vi "02.Evd.2_Ask.2.vi"() -> ()   [LabVIEW 2025]
panel:
  in  "Initial temperature in °C":dbl
  out "Kelvin":dbl
  out "Celsius":dbl
  out "Fahrenheit":dbl
  out "Kelvin":dbl(slide) scale=0.0..500.0
  out "Celsius":dbl(slide) scale=0.0..200.0
  out "Fahrenheit":dbl(slide) scale=0.0..300.0
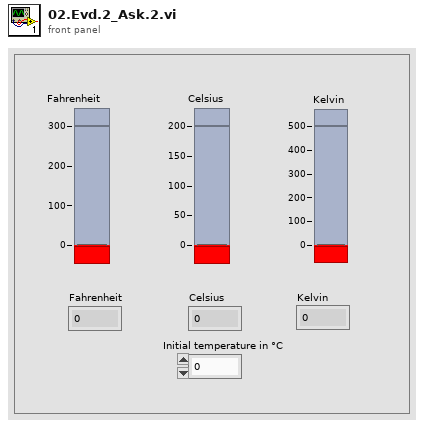
[diagram p1: front panel]
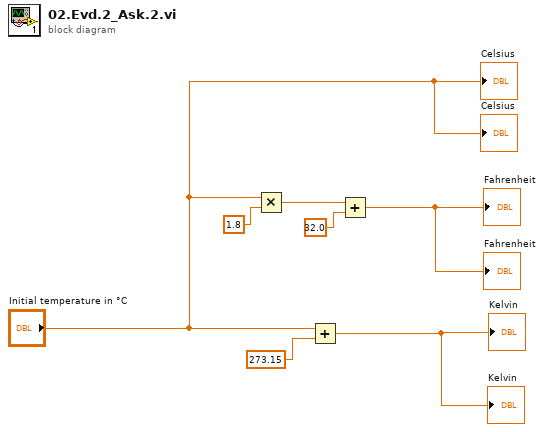
[diagram p0: block diagram]
diagram:
  n1 = Multiply(x="Initial temperature in °C", y=1.8) -> (x*y=w7:dbl)
  n2 = Add(x="Initial temperature in °C", y=273.15) -> (x+y=→"Kelvin" →"Kelvin":dbl)
  n3 = Add(x=w7, y=32.0) -> (x+y=→"Fahrenheit" →"Fahrenheit":dbl)
  "Celsius" <- "Initial temperature in °C"
  "Celsius" <- "Initial temperature in °C"
